vi "Write Specs URL.vi"(8 "error in (no error)":errorcluster, 10 "Specs URL":string, 11 "VI Package in":refnum<class "VIPM Package.lvclass">) -> (0 "error out":errorcluster, 3 "VI Package out":refnum<class "VIPM Package.lvclass">)   [LabVIEW 2016, in "Packages.lvlib" / "VIPM Package.lvclass"]
uses:
  VIPM Package.lvclass
  VIPM Package.lvclass/VIPM Package.ctl
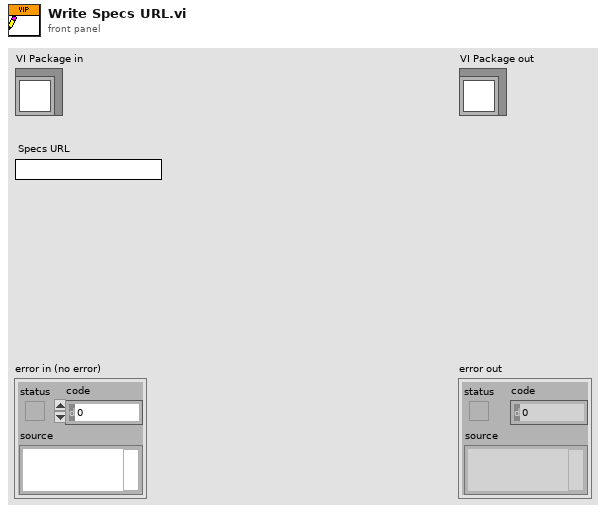
[diagram p1: front panel]
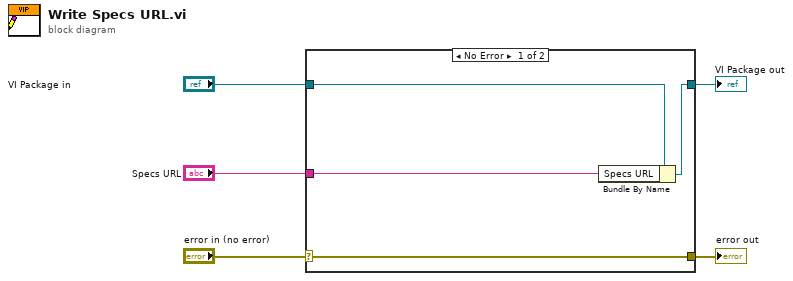
[diagram p0: block diagram]
diagram:
  n1 = case shown="No Error" "error in (no error)" {
    selector: "error in (no error)" -> [w9 w10]
    tunnel: [w9 w10] -> w4
    tunnel: [w7 w11] -> w2
    tunnel: "VI Package in" -> [w8 w11]
    tunnel: "Specs URL" -> [w6 _]
    frame No Error {
      n2 = Bundle By Name(cluster=w8, "Specs URL"=w6) -> (w7:refnum<class "VIPM Package.lvclass">)
    }
    frame Error {
    }
  }
  "error out" <- w4
  "VI Package out" <- w2
